vi "Bind RPC helloworld_Greeter_SayHello.vi"(11 "gRPCid server in":T3) -> (0 "error out":errorcluster, 1 "helloworld_Greeter_SayHello Internal UE":T2, 2 "helloworld_Greeter_SayHello gRPC UE":T1, 3 "gRPCid server out":T3)   [LabVIEW 2019, in "helloworld_server.lvlib" / "Greeter.lvclass"]
uses:
  Greeter.lvclass
  616620f9-6bbe-466a-af51-04bcc3596ea0.vi
  labview source/gRPC lv Support/grpc-lvsupport/grpcId.ctl
  labview source/gRPC lv Support/grpc-lvsupport/grpc-lvsupport.lvlib
  labview source/gRPC lv Support/grpc-lvsupport/gRPCId Cluster.ctl
  typeDefs/Server Internal Message.ctl
  typeDefs/Server Internal Message UE.ctl
  labview source/gRPC lv Support/grpc-lvsupport/gRPCId Cluster UE.ctl
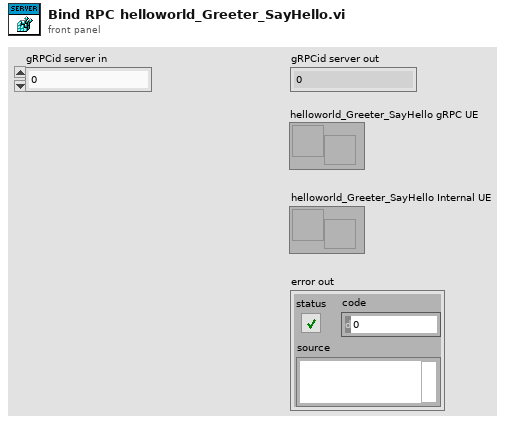
[diagram p1: front panel]
types:
  T1 = typedef "grpc-lvsupport.lvlib/gRPCId Cluster UE.ctl" = refnum<user-event>
  T2 = typedef "helloworld_server.lvlib/Greeter.lvclass/Server Internal Message UE.ctl" = refnum<user-event>
  T3 = typedef "grpc-lvsupport.lvlib/grpcId.ctl" = u64
  T4 = typedef "helloworld_server.lvlib/Greeter.lvclass/Server Internal Message.ctl" = cluster{"Command":string, "Data":variant}
  T5 = typedef "grpc-lvsupport.lvlib/gRPCId Cluster.ctl" = cluster{"gRPCid":T3}
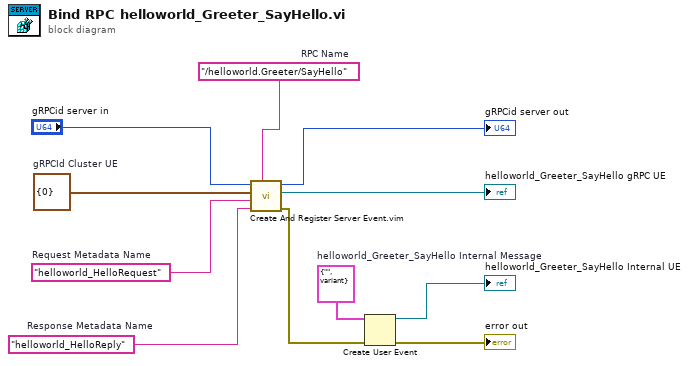
[diagram p0: block diagram]
diagram:
  w5 = T4 {"Command"="", "Data"=variant}  # helloworld_Greeter_SayHello Internal Message
  w8 = "helloworld_HelloReply"  # Response Metadata Name
  w11 = T5 {"gRPCid"=0}  # gRPCId Cluster UE
  w9 = "helloworld_HelloRequest"  # Request Metadata Name
  w10 = "/helloworld.Greeter/SayHello"  # RPC Name
  n1 = call "Create And Register Server Event.vim"("Method name"=w10, "Response Metadata Name"=w8, "Request Metadata Name"=w9, "event in"=w11, "gRPCid server in"="gRPCid server in") -> ("error out"=w4:errorcluster, "event"=→"helloworld_Greeter_SayHello gRPC UE":refnum<user-event>, "gRPCid server out"=→"gRPCid server out":T3)  [unwired: 4 in]
  n2 = Create User Event(user event datatype=w5, error in=w4) -> (user event=→"helloworld_Greeter_SayHello Internal UE":refnum<user-event>, error out=→"error out":errorcluster)
